vi "Vision Align.vi"(7 "VisionEnabled":bool, 11 "AngleEncoder":dbl) -> ()   [LabVIEW 2019]
uses:
  <vilib>/Rock Robotics/Network Tables/NT Read Numeric Array.vi
  Robot Global Data.vi
panel:
  in  "z-rotation factor":dbl=1.0 format="%#_13g"
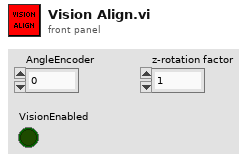
[diagram p1: front panel]
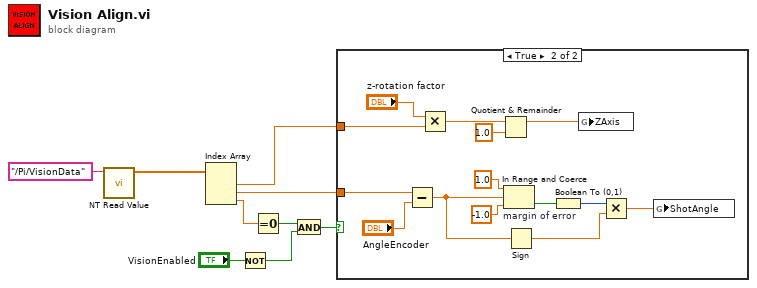
[diagram p0: block diagram]
diagram:
  n1 = call-poly <vilib>:"NT Read Value.vi"("Name"="/Pi/VisionData") -> ("Numeric Array"=w8:dbl[])  [unwired: 9 in, 1 out]
  n2 = Index Array(array=w8) -> (element #1=w6:dbl, element #2=w7:dbl, element #3=w5:dbl)  [unwired: 3 in]
  n3 = Not(x="VisionEnabled") -> (.not. x?=w1:bool)
  n4 = Equal To 0?(x=w5) -> (x = 0?=w4:bool)
  n5 = And(x=w4, y=w1) -> (x .and. y?=w3:bool)
  n6 = case shown="True" w3 {
    tunnel: w7 -> [_ w23]
    tunnel: w6 -> [_ w16]
    frame False {
    }
    frame True {
      n7 = Subtract(x=w23, y="AngleEncoder") -> (x-y=w13:dbl)
      n8 = Multiply(x="z-rotation factor", y=w16) -> (x*y=w12:dbl)
      n9 = Quotient & Remainder(x=w12, y=1.0) -> (x-y*floor(x/y)=w11:dbl)  [unwired: 1 out]
      n10 = In Range and Coerce "margin of error"(upper limit=1.0, x=w13, lower limit=-1.0) -> (In Range?=w19:bool)  [unwired: 1 out]
      n11 = Sign(1:w13) -> (0:w14:dbl)
      n12 = Boolean To (0,1)(Boolean=w19) -> (0, 1=w18:i16)
      n13 = global write "Robot Global Data.vi" "ZAxis"(w11) -> ()
      n14 = Multiply(x=w18, y=w14) -> (x*y=w15:dbl)
      n15 = global write "Robot Global Data.vi" "ShotAngle"(w15) -> ()
    }
  }
